vi "Create Queues.vi"(8 "Error In":errorcluster) -> (0 "Error Out":errorcluster)   [LabVIEW 2017]
uses:
  Reference Action.ctl
  Display Console/Communication/Display Console Queue Cluster.ctl
  Display Console/Communication/Display Console Message.ctl
  Controller/Communication/Controller Queue Message Cluster.ctl
  Controller/Communication/Controller Queue Message.ctl
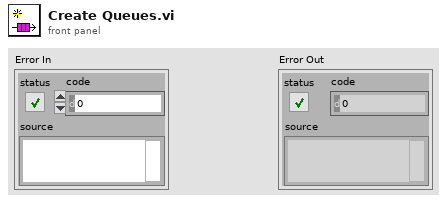
[diagram p1: front panel]
types:
  T1 = typedef "Controller Queue Message.ctl" = enum16{"Initialize", "User Console Update", "Sensor Update", "Wait for First Request", "Start and Move", "Analysis", "Continue Travel", "Stop at Floor", "Open and Close Door Sequence", "No Request Remaining", "Check Time", "Emergency Call", "Terminate Process", "Error Handling"}
  T2 = typedef "Display Console Message.ctl" = enum16{"Initialize", "Update", "Errror Handling", "Exit"}
  T3 = typedef "Controller Queue Message Cluster.ctl" = cluster{"Controller Queue Message":T1, "Controller Queue Data":variant}
  T4 = typedef "Display Console Queue Cluster.ctl" = cluster{"Display Console Message ":T2, "Display Console Data":variant}
  T5 = typedef "Reference Action.ctl" = enum16{"Set", "Get"}
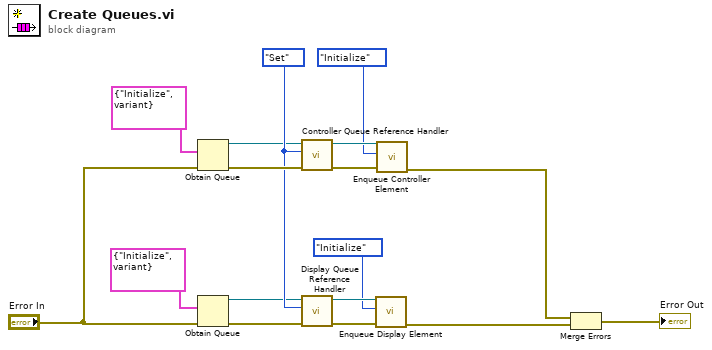
[diagram p0: block diagram]
diagram:
  w13 = Reference_Action."Set" ("Reference Action")
  n1 = Obtain Queue(element data type=T3 {"Controller Queue Message"=enum."Initialize", "Controller Queue Data"=variant} ("Controller Queue Cluster"), error in (no error)="Error In") -> (queue out=w10:refnum<queue>, error out=w17:errorcluster)  [unwired: 3 in, 1 out]
  n2 = Obtain Queue(element data type=T4 {"Display Console Message "=enum."Initialize", "Display Console Data"=variant} ("Display Console Queue Cluster"), error in (no error)="Error In") -> (queue out=w9:refnum<queue>, error out=w16:errorcluster)  [unwired: 3 in, 1 out]
  n3 = call "Controller Queue Reference Handler.vi"("Error In"=w17, "Reference Action"=w13, "Queue Ref In"=w10) -> ("Error Out"=w4:errorcluster, "Queue Ref Out"=w5:refnum<queue>)  [unwired: 7 in]
  n4 = call "Display Queue Reference Handler.vi"("Error In"=w16, "Reference Action"=w13, "Queue Ref In"=w9) -> ("Error Out"=w8:errorcluster, "Queue Ref Out"=w7:refnum<queue>)  [unwired: 7 in]
  n5 = call "Enqueue Display Element.vi"("error in (no error)"=w8, "Display Console Message"=Display_Console_Message."Initialize", "Message Queue"=w7) -> ("error out"=w2:errorcluster)  [unwired: 7 in, 1 out]
  n6 = call "Enqueue Controller Element.vi"("error in (no error)"=w4, "Controller Queue Message"=Controller_Queue_Message."Initialize", "Message Queue"=w5) -> ("error out"=w1:errorcluster)  [unwired: 7 in, 1 out]
  n7 = Merge Errors(w1, w2) -> (→"Error Out":errorcluster)
